vi "NF WF1973_74 RST.vi"(2 "Error In":errorcluster, 3 "VISAsession":refnum<visa-resource-name>) -> (0 "Error OUT":errorcluster, 1 "CopyVISAsession":refnum<visa-resource-name>)   [LabVIEW 2010]
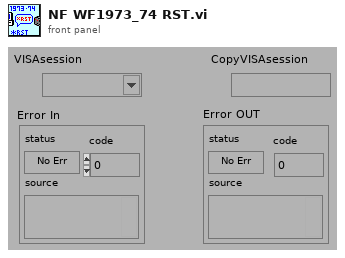
[diagram p1: front panel]
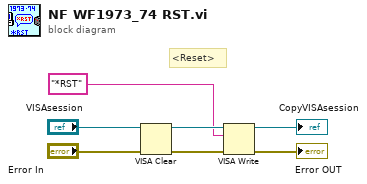
[diagram p0: block diagram]
diagram:
  # "<Reset>"
  n1 = VISA Clear(VISA resource name="VISAsession", error in (no error)="Error In") -> (VISA resource name out=w4:refnum<visa-resource-name>, error out=w3:errorcluster)
  n2 = VISA Write(VISA resource name=w4, write buffer="*RST", error in (no error)=w3) -> (VISA resource name out=→"CopyVISAsession":refnum<visa-resource-name>, error out=→"Error OUT":errorcluster)  [unwired: 1 out]
